vi "多参数关键参数读取.vi"(8 "Error in":errorcluster caption="Error in (no error)") -> (0 "error out":errorcluster, 3 "添加的数组":string[][](array[string]))   [LabVIEW 2016, in "斯坦道仪器.lvlib"]
panel:
  in  "关键参数区":i32(listbox)
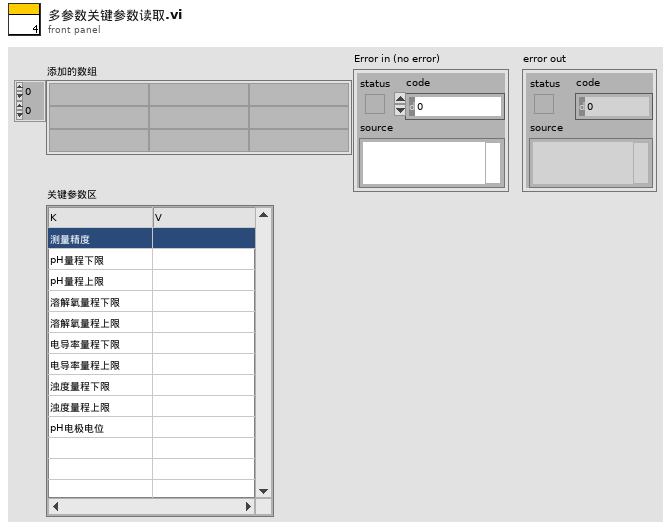
[diagram p1: front panel]
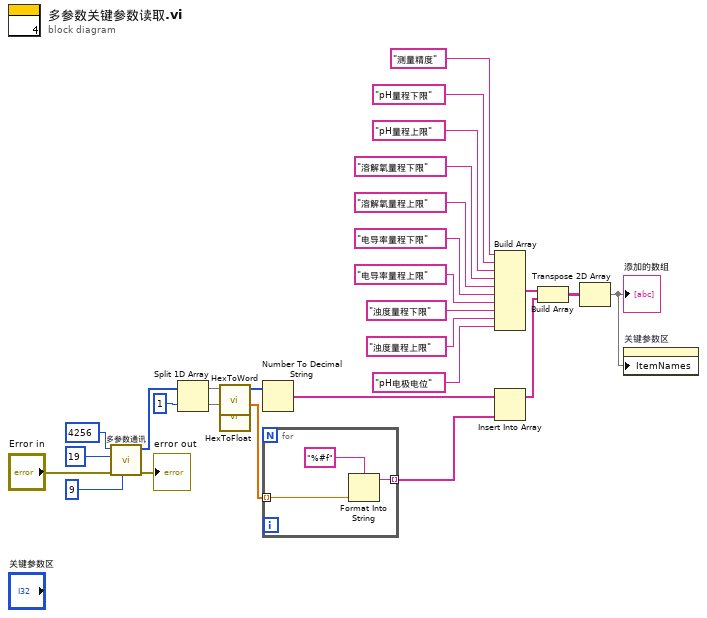
[diagram p0: block diagram]
diagram:
  n1 = call "多参数通讯.vi"("Slave ID"=u8 9, "Error in"="Error in", "quantity"=u16 19, "starting address"=u16 4256) -> ("error out"=→"error out":errorcluster, "Registers"=w25:u16[])  [unwired: 5 in, 1 out]
  n2 = Split 1D Array(array=w25, index=1 ("索引")) -> (first subarray=w11:u16[], second subarray=w10:u16[])
  n3 = call "HexToWord.vi"("数组"=w11) -> ("WORD"=w5:u16[])  [unwired: 10 in]
  n4 = call "HexToFloat.vi"("数组"=w10) -> ("FLOAT"=w3:sgl[])  [unwired: 10 in]
  n5 = Number To Decimal String(number=w5) -> (decimal integer string=w4:string[])  [unwired: 1 in]
  n6 = for {
    tunnel: w3 -> [w29] mode=indexing
    tunnel: [w28] -> w2 mode=indexing
    n7 = Format Into String(format string="%#f" ("格式字符串"), w29) -> (resulting string=w28:string)  [unwired: 2 in, 1 out]
  }
  n8 = Build Array("测量精度", "pH量程下限", "pH量程上限", "溶解氧量程下限", "溶解氧量程上限", "电导率量程下限", "电导率量程上限", "浊度量程下限", "浊度量程上限", "pH电极电位") -> (w13:string[])
  n9 = Insert Into Array(array=w4, new element=w2) -> (w9:string[])  [unwired: 1 in]
  n10 = Build Array(w13, w9) -> (w12:string[][])
  n11 = Transpose 2D Array(2D array=w12) -> (transposed array=w8:string[][])
  "添加的数组" <- w8
  n12 = property on="关键参数区" class="MCListbox (严格)"("ItemNames"=w8) -> ()  [unwired: 2 in, 2 out]
